vi "Heat1D_Cal Tridiagonal.vi"(9 "Boundary Condition":cluster{"type":T1, "Value":dbl[]}[](array[cluster]) {"type" items=["Dirichlet", "Neumann"]}, 10 "Coefficients":cluster{"r":dbl, "s":dbl, "dt":dbl, "dx":dbl}, 11 "Domain":T2) -> (1 "Super Diagonal":dbl[](array[numeric]), 2 "Main Diagonal":dbl[](array[numeric]), 3 "Sub Diagonal":dbl[](array[numeric]), 5 "Coeff Array":dbl[](array[numeric]))   [LabVIEW 2017, in "NI_PDE.lvlib"]
uses:
  <vilib>/gmath/NI_PDE.lvlib
  <vilib>/gmath/pde.llb/Common/PDE_BC Type.ctl
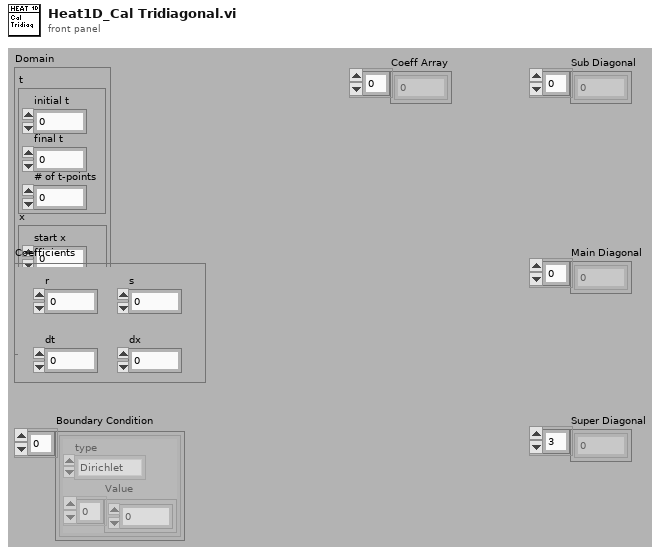
[diagram p1: front panel]
types:
  T1 = typedef "NI_PDE.lvlib/PDE_BC Type.ctl" = i32
  T2 = cluster{"t":cluster{"initial t":dbl, "final t":dbl, "# of t-points":i32}, "x":cluster{"start x":dbl, "end x":dbl, "# of x-points":i32}}
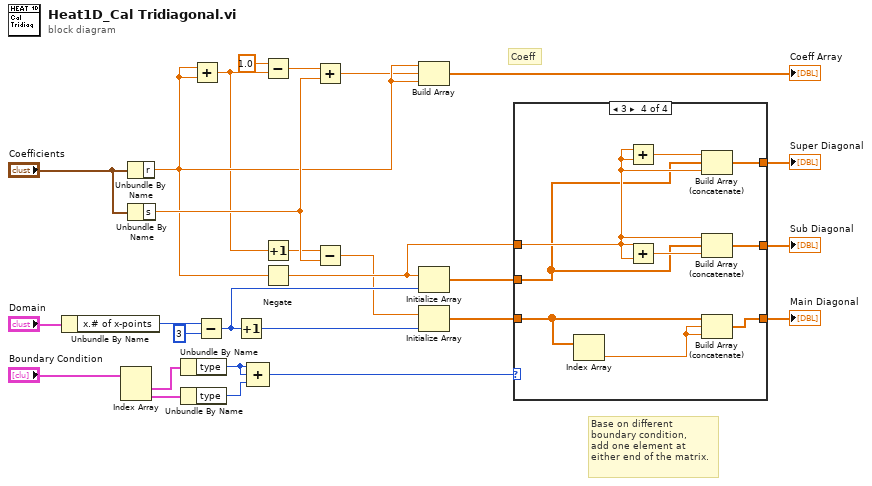
[diagram p0: block diagram]
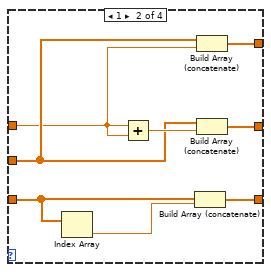
[diagram p3: hidden frame]
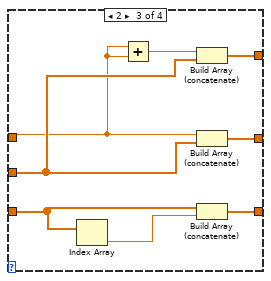
[diagram p4: hidden frame]
diagram:
  # "Coeff"
  # "Base on different \nboundary condition, \nadd one element at \neither end of the matrix."
  n1 = Unbundle By Name("Domain") -> ("x.# of x-points"=w22:i32)
  n2 = Index Array(array="Boundary Condition") -> (element #1=w20:cluster{"type":T1, "Value":dbl[]}, element #2=w19:cluster{"type":T1, "Value":dbl[]})  [unwired: 2 in]
  n3 = Unbundle By Name("Coefficients") -> ("r"=w24:dbl)
  n4 = Unbundle By Name("Coefficients") -> ("s"=w26:dbl)
  n5 = Unbundle By Name(w20) -> ("type"=w18:T1)
  n6 = Unbundle By Name(w19) -> ("type"=w17:T1)
  n7 = Add(x=w24, y=w24) -> (x+y=w1:dbl)
  n8 = Subtract(x=w22, y=3) -> (x-y=w9:i32)
  n9 = Increment(x=w9) -> (x+1=w10:i32)
  n10 = Compound Arithmetic op=ADD(w18, w18, w17) -> (w16:T1)
  n11 = Subtract(x=1.0, y=w1) -> (x-y=w5:dbl)
  n12 = Increment(x=w1) -> (x+1=w3:dbl)
  n13 = Negate(x=w24) -> (-x=w7:dbl)
  n14 = Add(x=w5, y=w26) -> (x+y=w4:dbl)
  n15 = Subtract(x=w3, y=w26) -> (x-y=w2:dbl)
  n16 = Build Array(w24, w4, w24) -> (→"Coeff Array":dbl[])
  n17 = Initialize Array(w7, w9) -> (w11:dbl[])
  n18 = Initialize Array(w2, w10) -> (w15:dbl[])
  n19 = case shown="3" w16 {
    tunnel: w15 -> [w29 w31 w45 w54]
    tunnel: [w29 w36 w43 w52] -> w14
    tunnel: w11 -> [w28 w32 w39 w46]
    tunnel: [w28 w35 w41 w50] -> w13
    tunnel: [w28 w33 w40 w48] -> w12
    tunnel: w7 -> [_ w30 w38 w47]
    frame 0, Default {
    }
    frame 1 {
      n20 = Index Array(array=w31) -> (element=w37:dbl)  [unwired: 1 in]
      n21 = Add(x=w30, y=w30) -> (x+y=w34:dbl)
      n22 = Build Array (concatenate)(w31, w37) -> (w36:dbl[])
      n23 = Build Array (concatenate)(w32, w30) -> (w35:dbl[])
      n24 = Build Array (concatenate)(w32, w34) -> (w33:dbl[])
    }
    frame 2 {
      n25 = Index Array(array=w45) -> (element=w44:dbl)  [unwired: 1 in]
      n26 = Add(x=w38, y=w38) -> (x+y=w42:dbl)
      n27 = Build Array (concatenate)(w42, w39) -> (w41:dbl[])
      n28 = Build Array (concatenate)(w38, w39) -> (w40:dbl[])
      n29 = Build Array (concatenate)(w45, w44) -> (w43:dbl[])
    }
    frame 3 {
      n30 = Index Array(array=w54) -> (element=w53:dbl)  [unwired: 1 in]
      n31 = Add(x=w47, y=w47) -> (x+y=w51:dbl)
      n32 = Add(x=w47, y=w47) -> (x+y=w49:dbl)
      n33 = Build Array (concatenate)(w51, w46, w47) -> (w50:dbl[])
      n34 = Build Array (concatenate)(w47, w46, w49) -> (w48:dbl[])
      n35 = Build Array (concatenate)(w54, w53, w53) -> (w52:dbl[])
    }
  }
  "Main Diagonal" <- w14
  "Super Diagonal" <- w13
  "Sub Diagonal" <- w12
